vi "000-Demo.vi"() -> ()   [LabVIEW 2019]
panel:
  out "?":bool
  out "?":bool
  out "?":bool
  out "Disciminant":dbl
  in  "c":dbl
  in  "b":dbl
  in  "a":dbl
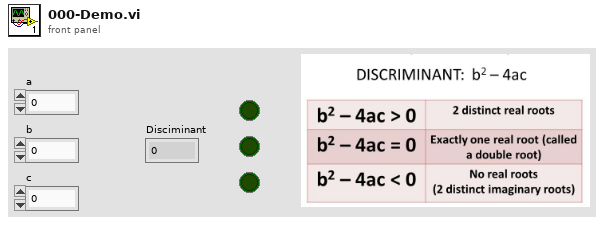
[diagram p1: front panel]
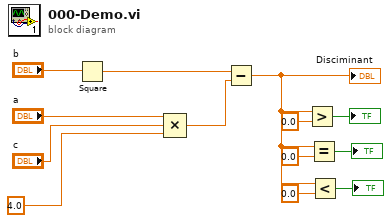
[diagram p0: block diagram]
diagram:
  n1 = Square(x="b") -> (x^2=w9:dbl)
  n2 = Compound Arithmetic op=MULTIPLY("a", "c", 4.0) -> (w8:dbl)
  n3 = Subtract(x=w9, y=w8) -> (x-y=w7:dbl)
  "Disciminant" <- w7
  n4 = Greater?(x=w7, y=0.0) -> (0:→"?":bool)
  n5 = Equal?(x=w7, y=0.0) -> (x = y?=→"?":bool)
  n6 = Less?(x=w7, y=0.0) -> (x < y?=→"?":bool)
